vi "Periodic Message Generator.vi"(0 "fgv references":T1, 5 "Output Array":T10[](array[typedef]) {"Identifier" format="%08x"}, 11 "error in":errorcluster) -> (6 "Output Array":T10[](array[typedef]) {"Identifier" format="%08x"}, 8 "Empty?":bool, 15 "error out":errorcluster)   [LabVIEW 2013, in "J1939.lvlib"]
uses:
  J1939.lvlib
  API Types/CAN Outgoing Message Cluster.ctl
  TP/TP List References.ctl
  BAM/BAM Buffer Connections List_Ref.ctl
  Connection Mode/Connection Mode Generation Connection Ref.ctl
  BAM/BAM Generation Connections List_Ref.ctl
  LUTs/J1939 Address Table Reference.ctl
  RQST/RQST Lookup Table Reference.ctl
  LUTs/J1939 Conversion Lookup Table Reference.ctl
  LUTs/J1939 Data Lookup Table Reference.ctl
  LUTs/Cyclic Frame Scheduler Lut Reference.ctl
  LUTs/Cyclic Frame Scheduler LUT Command.ctl
  Conversion Lookup Table Get Conversion Parameter.vi
  LUTs/J1939 Data Lookup Table Get Signals (Range).vi
  <vilib>/xnet/xnet.llb/XNET Convert.vi
  <vilib>/xnet/xnet.llb/XNET Convert (Signal to Frame Raw).vi
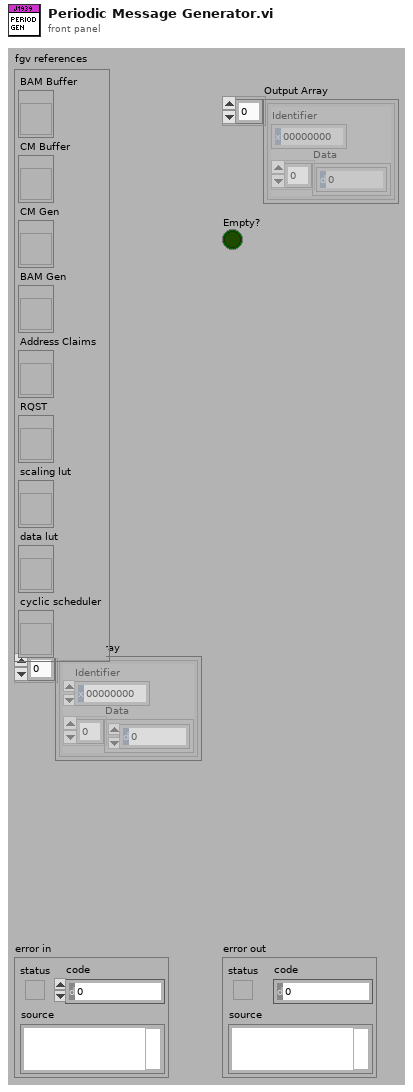
[diagram p1: front panel]
types:
  T1 = typedef "J1939.lvlib/TP List References.ctl" = cluster{"BAM Buffer":T2, "CM Buffer":T2, "CM Gen":T3, "BAM Gen":T4, "Address Claims":T5, "RQST":T6, "scaling lut":T7, "data lut":T8, "cyclic scheduler":T9}
  T2 = typedef "J1939.lvlib/BAM Buffer Connections List_Ref.ctl" = refnum<vi>
  T3 = typedef "J1939.lvlib/Connection Mode Generation Connection Ref.ctl" = refnum<vi>
  T4 = typedef "J1939.lvlib/BAM Generation Connections List_Ref.ctl" = refnum<vi>
  T5 = typedef "J1939.lvlib/J1939 Address Table Reference.ctl" = refnum<vi>
  T6 = typedef "J1939.lvlib/RQST Lookup Table Reference.ctl" = refnum<vi>
  T7 = typedef "J1939.lvlib/J1939 Conversion Lookup Table Reference.ctl" = refnum<vi>
  T8 = typedef "J1939.lvlib/J1939 Data Lookup Table Reference.ctl" = refnum<vi>
  T9 = typedef "J1939.lvlib/cyclic frame scheduler lut reference.ctl" = refnum<vi>
  T10 = typedef "J1939.lvlib/CAN Outgoing Message Cluster.ctl" = cluster{"Identifier":u32, "Data":u8[]}
  T11 = typedef "J1939.lvlib/cyclic frame scheduler lut command.ctl" = enum16{"Initialize", "set", "remove", "calculate times"}
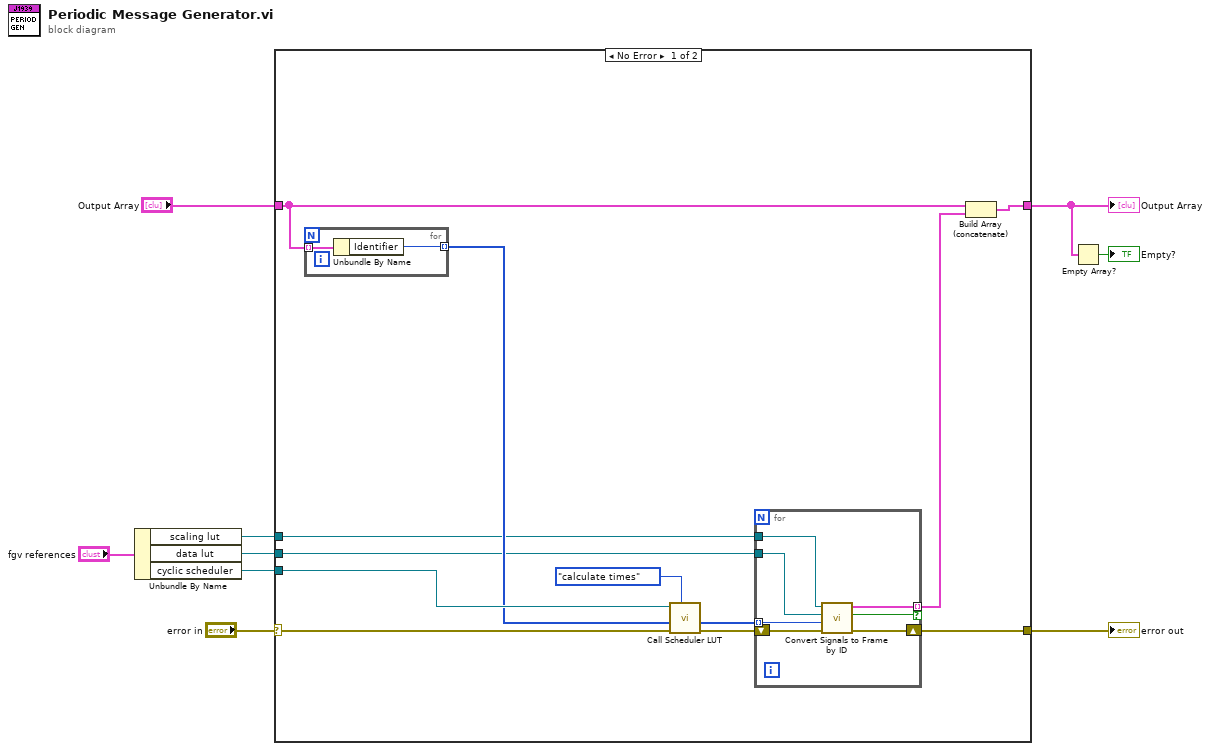
[diagram p0: block diagram]
diagram:
  n1 = Unbundle By Name("fgv references") -> ("scaling lut"=w4:T7, "data lut"=w3:T8, "cyclic scheduler"=w1:T9)
  n2 = case shown="No Error" "error in" {
    selector: "error in" -> [w21 w32]
    tunnel: [w14 w31] -> w6
    tunnel: [w16 w32] -> w8
    tunnel: "Output Array" -> [w15 w31]
    tunnel: w4 -> [w12 _]
    tunnel: w3 -> [w11 _]
    tunnel: w1 -> [w19 _]
    frame No Error {
      n3 = for {
        tunnel: w15 -> [w30] mode=indexing
        tunnel: [w29] -> w18 mode=indexing
        n4 = Unbundle By Name(w30) -> ("Identifier"=w29:u32)
      }
      n5 = call "Call Scheduler LUT.vi"("command"=cyclic_frame_scheduler_lut_command."calculate times", "error in"=w21, "pending frames"=w18, "scheduler lut"=w19) -> ("error out"=w17:errorcluster, "frames to generate"=w10:u32[])  [unwired: 6 in]
      n6 = for {
        shift-right: [w27] -> w16
        shift-left: w17 -> [w28]
        tunnel: [w26] -> w13 mode=indexing if=w25
        tunnel: w12 -> [w24]
        tunnel: w11 -> [w23]
        tunnel: w10 -> [w22] mode=indexing
        n7 = call "Convert Signals to Frame by ID.vi"("error in (no error)"=w28, "ID"=w22, "Data Ref"=w23, "Conv Ref"=w24) -> ("error out"=w27:errorcluster, "Found?"=w25:bool, "Frame"=w26:T10)  [unwired: 5 in]
      }
      n8 = Build Array (concatenate)(w15, w13) -> (w14:T10[])
    }
    frame Error {
    }
  }
  "error out" <- w8
  "Output Array" <- w6
  n9 = Empty Array?(array=w6) -> (empty?=→"Empty?":bool)
